vi "re_ClientSrv Tree Controller.vi"(0 "method":T2=enum."initialize", 5 "start path":path, 7 "tree control reference":refnum<vi>, 9 "pattern":string, 11 "file manipulation (local)":T1) -> ()   [LabVIEW 2012]
doc: "Initialises and populates a tree control with local or remote files and directories. This VI is reentrant so as to allow for parallel update of trees. The tags of each tree entry correspond to the path of the file or directory surrounded by double quotes."
uses:
  typedefs/t_ClientSrv Tree Controller Methods.ctl
  served/ClientSrv Server File Manipulation_srv.ctl
  typedefs/t_ClientSrv Tree Controller States.ctl
  typedefs/t_ClientSrv Server File Manipulation Methods.ctl
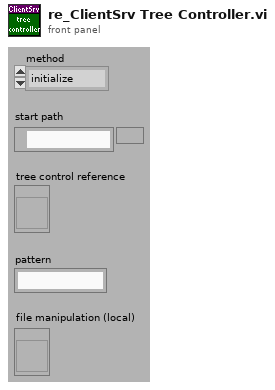
[diagram p1: front panel]
types:
  T1 = typedef "ClientSrv Server File Manipulation_srv.ctl" = refnum<vi>
  T2 = typedef "t_ClientSrv Tree Controller Methods.ctl" = enum16{"do nothing", "initialize", "open item", "close item", "refresh"}
  T3 = typedef "t_ClientSrv Tree Controller States.ctl" = enum16{"initialize", "init roots", "reinit roots", "open item", "close item", "populate", "readjust", "refresh", "stop"}
  T4 = typedef "t_ClientSrv Server File Manipulation Methods.ctl" = enum16{"close", "list", "open", "new", "read", "write", "newdir", "info", "rename", "delete"}
  T5 = typedef "LVNodeAndColumnTypeDef.ctl" = cluster{"Node":string, "Column":i32}
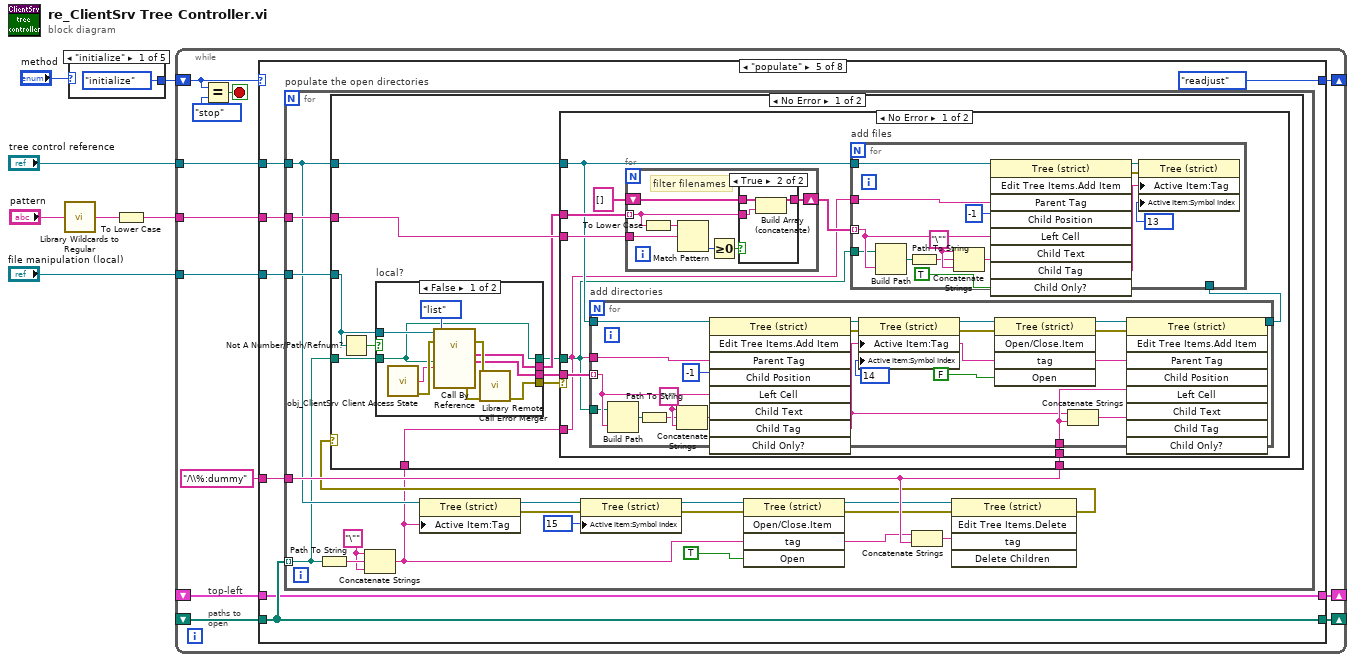
[diagram p0: block diagram]
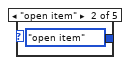
[diagram p2: hidden frame]
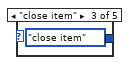
[diagram p3: hidden frame]
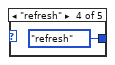
[diagram p4: hidden frame]
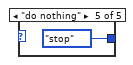
[diagram p5: hidden frame]
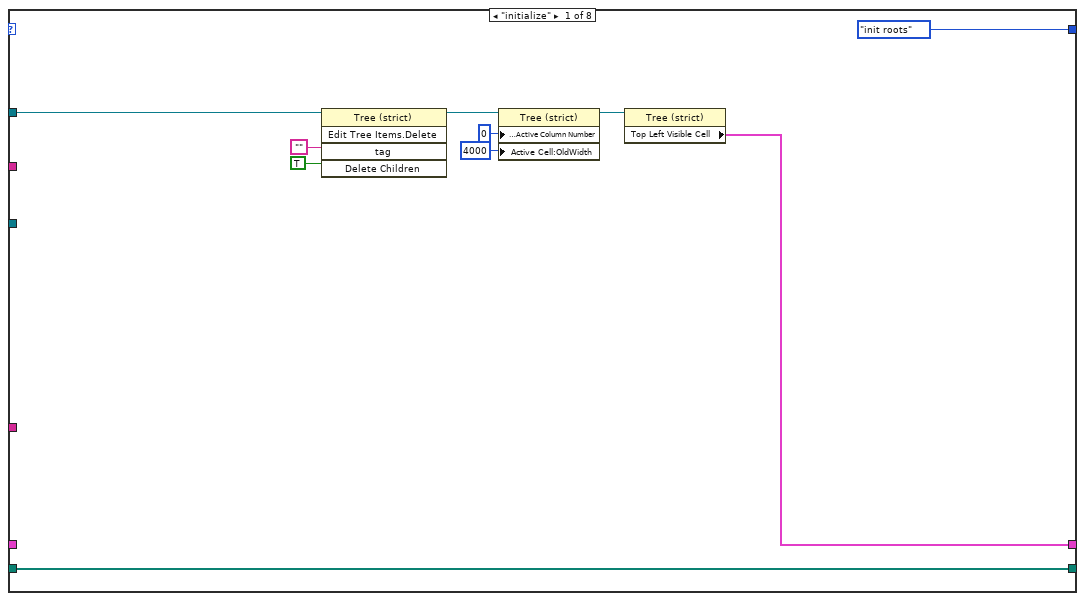
[diagram p6: hidden frame]
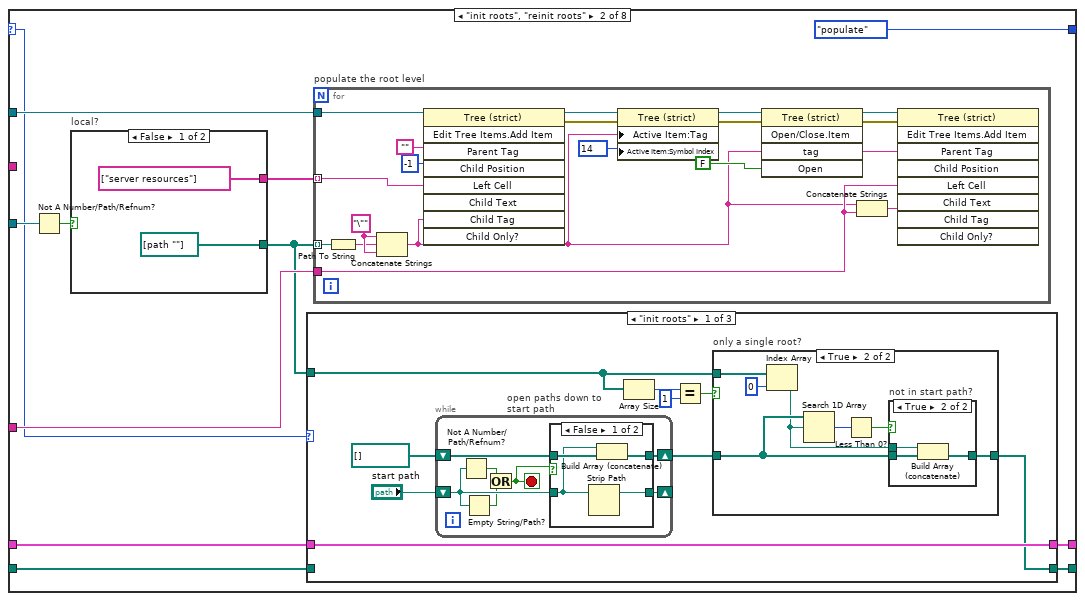
[diagram p7: hidden frame]
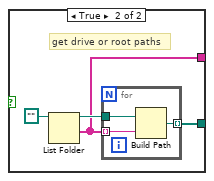
[diagram p13: hidden frame]
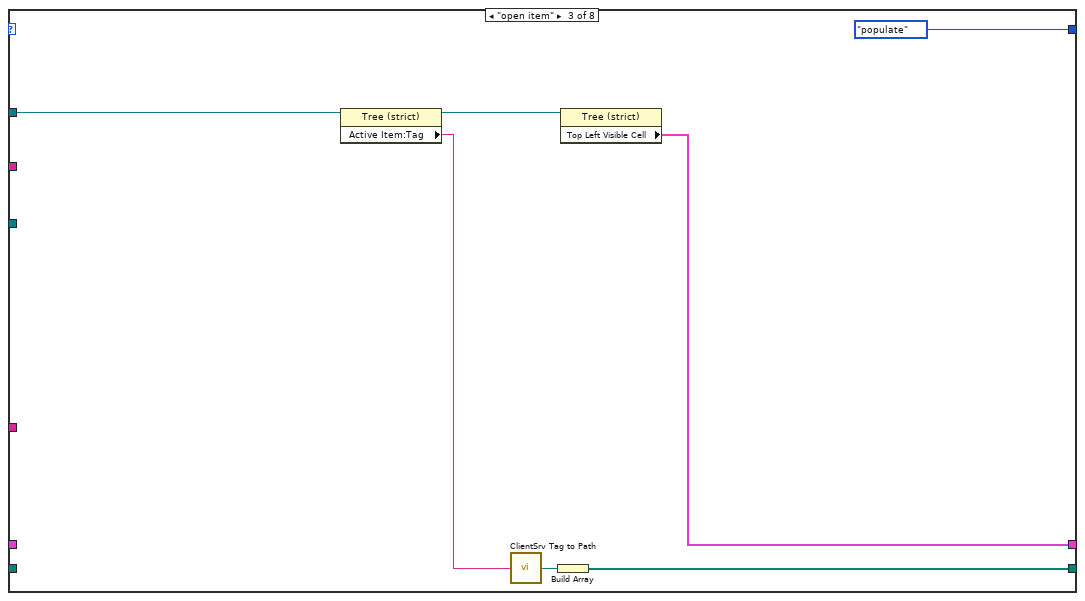
[diagram p14: hidden frame]
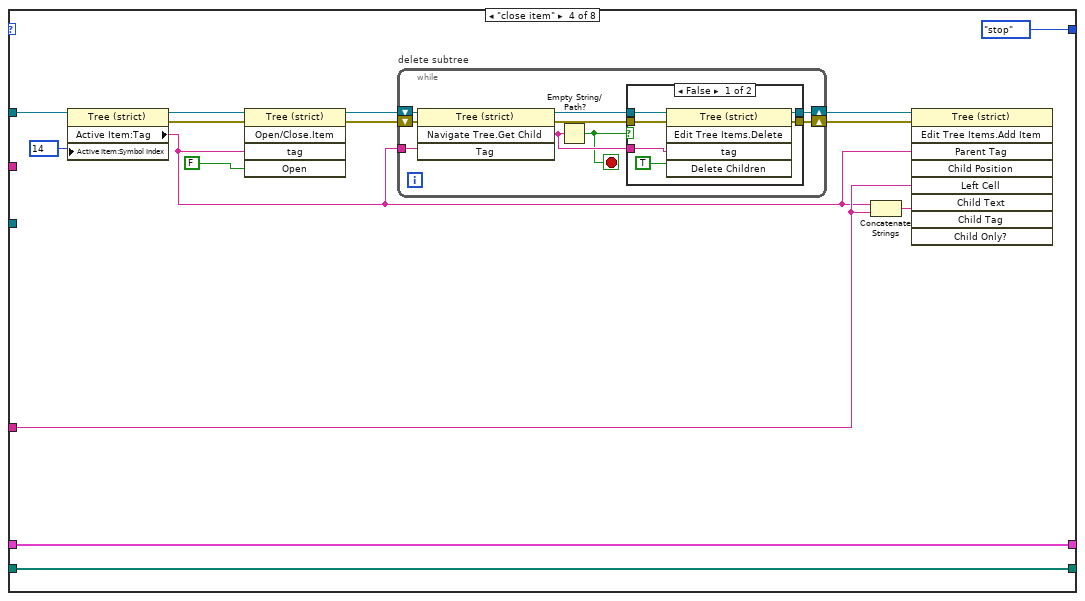
[diagram p15: hidden frame]
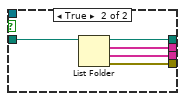
[diagram p17: hidden frame]
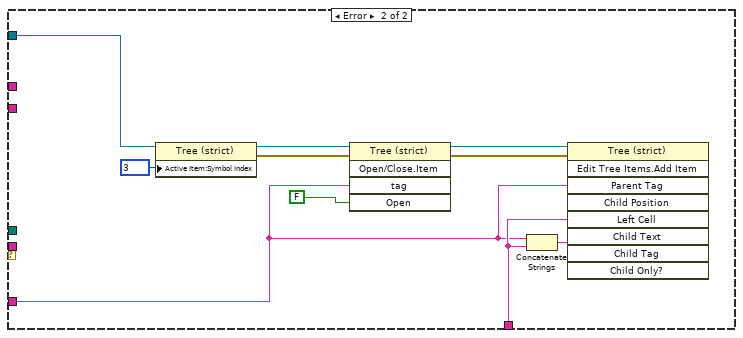
[diagram p19: hidden frame]
diagram:
  n1 = call "Library Wildcards to Regular.vi"("wildcards"="pattern") -> ("regular expression"=w1:string)  [unwired: 4 in]
  n2 = case shown="\"initialize\"" "method" {
    tunnel: [t_ClientSrv_Tree_Controller_States."initialize" ("y") t_ClientSrv_Tree_Controller_States."open item" ("y") t_ClientSrv_Tree_Controller_States."close item" ("y") t_ClientSrv_Tree_Controller_States."refresh" ("y") t_ClientSrv_Tree_Controller_States."stop" ("y")] -> w4
    frame "initialize" {
    }
    frame "open item" {
    }
    frame "close item" {
    }
    frame "refresh" {
    }
    frame "do nothing" {
    }
  }
  n3 = To Lower Case(string=w1) -> (all lower case string=w3:string)
  n4 = while {
    shift-right: [w24] -> _
    shift-left: _ -> [w23]
    shift-right: [w22] -> _
    shift-left: _ -> [w21]
    shift-right: [w17] -> _
    shift-left: w4 -> [w18]
    tunnel: w3 -> [w16]
    tunnel: "tree control reference" -> [w15]
    tunnel: "file manipulation (local)" -> [w13]
    stop <- w19 stop-if-true
    # "top-left"
    # "paths to open"
    n5 = Equal?(x=w18, y=t_ClientSrv_Tree_Controller_States."stop") -> (x = y?=w19:bool)
    n6 = case shown="\"populate\"" w18 {
      selector: w18 -> [_ w35 _ _ _ _ _ w330]
      tunnel: w16 -> [_ _ _ _ w157 _ _ _]
      tunnel: w15 -> [w34 w46 w118 w130 w156 w271 w280 _]
      tunnel: [w26 w38 w117 w132 w153 w272 w286 w331] -> w22
      tunnel: [w28 w40 w115 w133 w155 w274 w283 w332] -> w24
      tunnel: w23 -> [w28 w37 _ w133 w155 w274 _ w332]
      tunnel: w21 -> [_ w39 _ w132 w153 w272 _ w331]
      tunnel: [t_ClientSrv_Tree_Controller_States."init roots" ("y") t_ClientSrv_Tree_Controller_States."populate" ("y") t_ClientSrv_Tree_Controller_States."populate" ("y") t_ClientSrv_Tree_Controller_States."stop" ("y") t_ClientSrv_Tree_Controller_States."readjust" ("y") t_ClientSrv_Tree_Controller_States."stop" ("y") t_ClientSrv_Tree_Controller_States."reinit roots" ("y") w330] -> w17
      tunnel: "/\\%:dummy" ("Left Cell String") -> [_ w41 _ w127 w152 _ _ _]
      tunnel: w13 -> [_ w44 _ _ w151 _ _ _]
      frame "initialize" {
        n7 = invoke on="Invoke Node" class="Tree (strict)" method="Edit Tree Items.Delete"(reference=w34, "tag"="", "Delete Children"=TRUE) -> (reference out=w25:refnum<vi>)  [unwired: 2 in, 4 out]
        n8 = property on="Property Node" class="Tree (strict)"(reference=w25, "Active Cell:Active Column Number"=0 ("Active Cell Properties:Active Column Number"), "Active Cell:OldWidth"=4000 ("Active Cell Properties:Cell Size:Width")) -> (reference out=w27:refnum<vi>)  [unwired: 1 in, 1 out]
        n9 = property on="Property Node" class="Tree (strict)"(reference=w27) -> ("Top Left Visible Cell"=w26:T5)  [unwired: 1 in, 2 out]
      }
      frame "init roots", "reinit roots" {
        n10 = Not A Number/Path/Refnum?(number/path/refnum=w44) -> (NaN/Path/Refnum?=w42:bool)
        n11 = case "local?" shown="False" w42 {
          tunnel: [path[] [path ""] w88] -> w36
          tunnel: [string[] ["server resources"] w87] -> w43
          frame False {
          }
          frame True {
            # "get drive or root paths"
            n12 = List Folder(path=path "") -> (path out=w90:path, folder names=w87:string[])  [unwired: 3 in, 2 out]
            n13 = for {
              tunnel: w90 -> [w93]
              tunnel: w87 -> [w91] mode=indexing
              tunnel: [w92] -> w88 mode=indexing
              n14 = Build Path(base path=w93, name or relative path=w91) -> (appended path=w92:path)
            }
          }
        }
        n15 = case shown="\"init roots\"" w35 {
          tunnel: [w48 w81 w83] -> w40
          tunnel: w39 -> [w52 w82 w84]
          tunnel: [w52 w82 w84] -> w38
          tunnel: w37 -> [_ w81 w83]
          tunnel: w36 -> [w51 _ _]
          frame "init roots" {
            n16 = while "open paths down to start path" {
              shift-right: [w62] -> _
              shift-left: "start path" -> [w59]
              shift-right: [w60] -> w49
              shift-left: path[] [] -> [w61]
              stop <- w56 stop-if-true
              n17 = Not A Number/Path/Refnum?(number/path/refnum=w59) -> (NaN/Path/Refnum?=w58:bool)
              n18 = Empty String/Path?(string/path=w59) -> (empty?=w57:bool)
              n19 = Or(x=w58, y=w57) -> (x .or. y?=w56:bool)
              n20 = case shown="False" w56 {
                tunnel: w59 -> [w64 w68]
                tunnel: [w66 w68] -> w62
                tunnel: w61 -> [w65 w67]
                tunnel: [w63 w67] -> w60
                frame False {
                  n21 = Strip Path(path=w64) -> (stripped path=w66:path)  [unwired: 1 out]
                  n22 = Build Array (concatenate)(w64, w65) -> (w63:path[])
                }
                frame True {
                }
              }
            }
            n23 = Array Size(array=w51) -> (size(s)=w55:i32)
            n24 = Equal?(x=w55, y=1) -> (x = y?=w53:bool)
            n25 = case "only a single root?" shown="True" w53 {
              tunnel: w51 -> [_ w76]
              tunnel: w49 -> [w69 w72]
              tunnel: [w69 w71] -> w48
              frame False {
              }
              frame True {
                n26 = Index Array(array=w76, index=0) -> (element=w70:path)
                n27 = Search 1D Array(1D array=w72, element=w70) -> (index of element=w74:i32)  [unwired: 1 in]
                n28 = Less Than 0?(x=w74) -> (x < 0?=w73:bool)
                n29 = case "not in start path?" shown="True" w73 {
                  tunnel: w72 -> [w77 w80]
                  tunnel: [w77 w79] -> w71
                  tunnel: w70 -> [_ w78]
                  frame False {
                  }
                  frame True {
                    n30 = Build Array (concatenate)(w78, w80) -> (w79:path[])
                  }
                }
              }
            }
          }
          frame "reinit roots" {
          }
          frame Default {
            # "never happens"
          }
        }
        n31 = for "populate the root level" {
          tunnel: w46 -> [w111]
          tunnel: w36 -> [w95] mode=indexing
          tunnel: w43 -> [w101] mode=indexing
          tunnel: w41 -> [w99]
          w97 = "\"" ("string")
          n32 = Path To String(path=w95) -> (string=w96:string)
          n33 = Concatenate Strings(w97, w96, w97) -> (w94:string)
          n34 = invoke class="Tree (strict)" method="Edit Tree Items.Add Item"(reference=w111, "Parent Tag"="", "Child Position"=-1, "Left Cell"=w101, "Child Tag"=w94) -> (reference out=w110:refnum<vi>, error out=w108:errorcluster)  [unwired: 4 in, 7 out]
          n35 = property class="Tree (strict)"(reference=w110, error in=w108, "Active Item:Tag"=w94, "Active Item:Symbol Index"=14) -> (reference out=w107:refnum<vi>, error out=w106:errorcluster)
          n36 = invoke class="Tree (strict)" method="Open/Close.Item"(reference=w107, error in=w106, "tag"=w94, "Open"=FALSE) -> (reference out=w105:refnum<vi>, error out=w104:errorcluster)  [unwired: 1 in, 3 out]
          n37 = Concatenate Strings(w94, w99) -> (w103:string)
          n38 = invoke class="Tree (strict)" method="Edit Tree Items.Add Item"(reference=w105, error in=w104, "Parent Tag"=w94, "Left Cell"=w99, "Child Tag"=w103) -> ()  [unwired: 4 in, 9 out]
        }
      }
      frame "open item" {
        n39 = property on="Property Node" class="Tree (strict)"(reference=w118) -> (reference out=w112:refnum<vi>, "Active Item:Tag"=w113:string)  [unwired: 1 in, 1 out]
        n40 = call "ClientSrv Tag to Path.vi"("tree tag"=w113) -> ("path"=w114:path)
        n41 = Build Array(w114) -> (w115:path[])
        n42 = property on="Property Node" class="Tree (strict)"(reference=w112) -> ("Top Left Visible Cell"=w117:T5)  [unwired: 1 in, 2 out]
      }
      frame "close item" {
        n43 = property class="Tree (strict)"(reference=w130, "Active Item:Symbol Index"=14) -> (reference out=w124:refnum<vi>, error out=w121:errorcluster, "Active Item:Tag"=w120:string)  [unwired: 1 in]
        n44 = invoke on="Invoke Node" class="Tree (strict)" method="Open/Close.Item"(reference=w124, error in=w121, "tag"=w120, "Open"=FALSE) -> (reference out=w123:refnum<vi>, error out=w122:errorcluster)  [unwired: 1 in, 3 out]
        n45 = while "delete subtree" {
          tunnel: w120 -> [w141]
          shift-right: [w137] -> w129
          shift-left: w123 -> [w142]
          shift-right: [w134] -> w125
          shift-left: w122 -> [w136]
          stop <- w138 stop-if-true
          n46 = invoke on="Invoke Node" class="Tree (strict)" method="Navigate Tree.Get Child"(reference=w142, error in=w136, "Tag"=w141) -> (reference out=w140:refnum<vi>, error out=w135:errorcluster, "Navigate Tree:Get Child"=w139:string)  [unwired: 1 in, 1 out]
          n47 = Empty String/Path?(string/path=w139) -> (empty?=w138:bool)
          n48 = case shown="False" w138 {
            tunnel: w140 -> [w148 w150]
            tunnel: w139 -> [w147 _]
            tunnel: [w145 w150] -> w137
            tunnel: w135 -> [w144 w149]
            tunnel: [w143 w149] -> w134
            frame False {
              n49 = invoke on="Invoke Node" class="Tree (strict)" method="Edit Tree Items.Delete"(reference=w148, error in=w144, "tag"=w147, "Delete Children"=TRUE) -> (reference out=w145:refnum<vi>, error out=w143:errorcluster)  [unwired: 1 in, 3 out]
            }
            frame True {
            }
          }
        }
        n50 = Concatenate Strings(w120, w127) -> (w128:string)
        n51 = invoke class="Tree (strict)" method="Edit Tree Items.Add Item"(reference=w129, error in=w125, "Parent Tag"=w120, "Left Cell"=w127, "Child Tag"=w128) -> ()  [unwired: 4 in, 9 out]
      }
      frame "populate" {
        n52 = for "populate the open directories" {
          tunnel: w155 -> [w160] mode=indexing
          tunnel: w157 -> [w175]
          tunnel: w156 -> [w167]
          tunnel: w152 -> [w174]
          tunnel: w151 -> [w173]
          w161 = "\"" ("string")
          n53 = Path To String(path=w160) -> (string=w162:string)
          n54 = Concatenate Strings(w161, w162, w161) -> (w159:string)
          n55 = property on="Property Node" class="Tree (strict)"(reference=w167, "Active Item:Tag"=w159) -> (reference out=w166:refnum<vi>, error out=w158:errorcluster)  [unwired: 1 in]
          n56 = property on="Property Node" class="Tree (strict)"(reference=w166, error in=w158, "Active Item:Symbol Index"=15) -> (reference out=w165:refnum<vi>, error out=w164:errorcluster)
          n57 = invoke on="Invoke Node" class="Tree (strict)" method="Open/Close.Item"(reference=w165, error in=w164, "tag"=w159, "Open"=TRUE ("Delete Children")) -> (reference out=w172:refnum<vi>, error out=w169:errorcluster)  [unwired: 1 in, 3 out]
          n58 = Concatenate Strings(w159, w174) -> (w171:string)
          n59 = invoke on="Invoke Node" class="Tree (strict)" method="Edit Tree Items.Delete"(reference=w172, error in=w169, "tag"=w171) -> (error out=w168:errorcluster)  [unwired: 2 in, 4 out]
          n60 = case shown="No Error" w168 {
            tunnel: w160 -> [w186 _]
            tunnel: w175 -> [w185 _]
            tunnel: w167 -> [w184 _]
            tunnel: w174 -> [w183 _]
            tunnel: w173 -> [w181 _]
            tunnel: w159 -> [w176 _]
            frame No Error {
              n61 = Not A Number/Path/Refnum?(number/path/refnum=w181) -> (NaN/Path/Refnum?=w182:bool)
              n62 = case "local?" shown="False" w182 {
                tunnel: w186 -> [w192 w201]
                tunnel: [w191 w200] -> w180
                tunnel: [w188 w199] -> w179
                tunnel: [w187 w198] -> w178
                tunnel: [w192 w197] -> w177
                tunnel: w181 -> [w195 _]
                frame False {
                  n63 = call "obj_ClientSrv Client Access State.vi"() -> ("certificate"=w193:string, "error out"=w196:errorcluster)  [unwired: 14 in]
                  n64 = call-by-ref "?"(reference=w195, error in=w196, "method"=t_ClientSrv_Server_File_Manipulation_Methods."list", "path"=w192, "certificate"=w193) -> (error out=w190:errorcluster, "file names"=w188:string[], "directory names"=w187:string[], 15:"error out"=w189:errorcluster)  [unwired: 5 in, 6 out]
                  n65 = call "Library Remote Call Error Merger.vi"("call by reference node error"=w190, "called VI error (no error)"=w189) -> ("error out"=w191:errorcluster)  [unwired: 13 in]
                }
                frame True {
                  n66 = List Folder(path=w201) -> (path out=w197:path, filenames=w199:string[], folder names=w198:string[], error out=w200:errorcluster)  [unwired: 3 in]
                }
              }
              n67 = case shown="No Error" w180 {
                tunnel: w178 -> [w211 _]
                tunnel: w177 -> [w203 _]
                tunnel: w184 -> [w205 w265]
                tunnel: w185 -> [w207 _]
                tunnel: w179 -> [w209 _]
                tunnel: w183 -> [w204 w258]
                tunnel: w176 -> [w202 w256]
                frame No Error {
                  n68 = for "add directories" {
                    tunnel: w203 -> [w244]
                    tunnel: w211 -> [w254] mode=indexing
                    tunnel: w205 -> [w251]
                    tunnel: [w242] -> w206
                    tunnel: w204 -> [w241]
                    tunnel: w202 -> [w236]
                    w240 = "\"" ("string")
                    n69 = Build Path(base path=w244, name or relative path=w254) -> (appended path=w237:path)
                    n70 = Path To String(path=w237) -> (string=w238:string)
                    n71 = Concatenate Strings(w240, w238, w240) -> (w239:string)
                    n72 = invoke on="Invoke Node" class="Tree (strict)" method="Edit Tree Items.Add Item"(reference=w251, "Parent Tag"=w236, "Child Position"=-1 ("Child Posn"), "Left Cell"=w254, "Child Tag"=w239) -> (reference out=w250:refnum<vi>, error out=w252:errorcluster)  [unwired: 4 in, 7 out]
                    n73 = property on="Property Node" class="Tree (strict)"(reference=w250, error in=w252, "Active Item:Tag"=w239, "Active Item:Symbol Index"=14) -> (reference out=w249:refnum<vi>, error out=w243:errorcluster)
                    n74 = invoke class="Tree (strict)" method="Open/Close.Item"(reference=w249, error in=w243, "tag"=w239, "Open"=FALSE) -> (reference out=w247:refnum<vi>, error out=w246:errorcluster)  [unwired: 1 in, 3 out]
                    n75 = Concatenate Strings(w239, w241) -> (w245:string)
                    n76 = invoke class="Tree (strict)" method="Edit Tree Items.Add Item"(reference=w247, error in=w246, "Parent Tag"=w239, "Left Cell"=w241, "Child Tag"=w245) -> (reference out=w242:refnum<vi>)  [unwired: 4 in, 8 out]
                  }
                  n77 = for {
                    tunnel: w209 -> [w216] mode=indexing
                    shift-right: [w214] -> w208
                    shift-left: string[] [] -> [w215]
                    tunnel: w207 -> [w213]
                    # "filter filenames"
                    n78 = To Lower Case(string=w216) -> (all lower case string=w212:string)
                    n79 = Match Pattern(string=w212, regular expression=w213) -> (offset past match=w218:i32)  [unwired: 1 in, 3 out]
                    n80 = Greater Or Equal To 0?(x=w218) -> (x >= 0?=w217:bool)
                    n81 = case shown="True" w217 {
                      tunnel: w216 -> [_ w222]
                      tunnel: w215 -> [w219 w221]
                      tunnel: [w219 w220] -> w214
                      frame False {
                      }
                      frame True {
                        n82 = Build Array (concatenate)(w221, w222) -> (w220:string[])
                      }
                    }
                  }
                  n83 = for "add files" {
                    tunnel: w203 -> [w232]
                    tunnel: w208 -> [w234] mode=indexing
                    tunnel: w205 -> [w229]
                    tunnel: w206 -> [_]
                    tunnel: w202 -> [w223]
                    w227 = "\"" ("string")
                    n84 = Build Path(base path=w232, name or relative path=w234) -> (appended path=w225:path)
                    n85 = Path To String(path=w225) -> (string=w226:string)
                    n86 = Concatenate Strings(w227, w226, w227) -> (w224:string)
                    n87 = invoke on="Invoke Node" class="Tree (strict)" method="Edit Tree Items.Add Item"(reference=w229, "Parent Tag"=w223, "Child Position"=-1 ("Child Posn"), "Left Cell"=w234, "Child Tag"=w224, "Child Only?"=TRUE) -> (reference out=w228:refnum<vi>, error out=w231:errorcluster)  [unwired: 3 in, 7 out]
                    n88 = property on="Property Node" class="Tree (strict)"(reference=w228, error in=w231, "Active Item:Tag"=w224, "Active Item:Symbol Index"=13) -> ()  [unwired: 2 out]
                  }
                }
                frame Error {
                  n89 = property on="Property Node" class="Tree (strict)"(reference=w265, "Active Item:Symbol Index"=3) -> (reference out=w263:refnum<vi>, error out=w262:errorcluster)  [unwired: 1 in]
                  n90 = invoke on="Invoke Node" class="Tree (strict)" method="Open/Close.Item"(reference=w263, error in=w262, "tag"=w256, "Open"=FALSE) -> (reference out=w259:refnum<vi>, error out=w257:errorcluster)  [unwired: 1 in, 3 out]
                  n91 = Concatenate Strings(w256, w258) -> (w260:string)
                  n92 = invoke class="Tree (strict)" method="Edit Tree Items.Add Item"(reference=w259, error in=w257, "Parent Tag"=w256, "Left Cell"=w258, "Child Tag"=w260) -> ()  [unwired: 4 in, 9 out]
                }
              }
            }
            frame Error {
            }
          }
        }
      }
      frame "readjust" {
        n93 = property on="Property Node" class="Tree (strict)"(reference=w271) -> (reference out=w270:refnum<vi>, "Value"=w269:string)  [unwired: 1 in, 1 out]
        n94 = property on="Property Node" class="Tree (strict)"(reference=w270, "Active Item:Tag"=w269) -> (reference out=w267:refnum<vi>, error out=w268:errorcluster)  [unwired: 1 in]
        n95 = case "selected item still present?" shown="Error" w268 {
          tunnel: w267 -> [w275 w278]
          tunnel: [w275 w277] -> w266
          frame No Error {
          }
          frame Error {
            n96 = property on="Property Node" class="Tree (strict)"(reference=w278, "Value"="") -> (reference out=w277:refnum<vi>)  [unwired: 1 in, 1 out]
          }
        }
        n97 = property on="Property Node" class="Tree (strict)"(reference=w266, "Top Left Visible Cell"=w272) -> ()  [unwired: 1 in, 2 out]
      }
      frame "refresh" {
        w287 = string[] []
        n98 = property on="Property Node" class="Tree (strict)"(reference=w280) -> (reference out=w285:refnum<vi>, "Top Left Visible Cell"=w286:T5)  [unwired: 1 in, 1 out]
        n99 = while "traverse tree breadth-first to determine the open directories" {
          shift-right: [w298] -> _
          shift-left: "" -> [w293]
          shift-right: [w305] -> w284
          shift-left: w287 -> [w306]
          shift-right: [w303] -> _
          shift-left: w287 -> [w304]
          shift-right: [w297] -> w281
          shift-left: w285 -> [w297]
          stop <- w299 stop-if-true
          # "open directories to traverse"
          # "open directories"
          n100 = property on="Property Node" class="Tree (strict)"(reference=w297, "Active Item:Tag"=w293) -> (reference out=w296:refnum<vi>, "Active Item:Open?"=w294:bool, "Active Item:Child-Only?"=w295:bool)  [unwired: 1 in, 1 out]
          n101 = Empty String/Path?(string/path=w293) -> (empty?=w291:bool)
          n102 = Compound Arithmetic op=AND(w294, invert w295, invert w291) -> (w292:bool)
          n103 = case "open directory?" shown="False" w292 {
            tunnel: w306 -> [w313 w329]
            tunnel: w293 -> [w311 w325]
            tunnel: [w313 w328] -> w305
            tunnel: w304 -> [w312 w327]
            tunnel: [w310 w324] -> w298
            tunnel: [w309 w326] -> w303
            tunnel: w296 -> [w308 w323]
            tunnel: w291 -> [w307 _]
            frame False {
              n104 = case shown="True" w307 {
                tunnel: w312 -> [w317 w322]
                tunnel: [w315 w320] -> w310
                tunnel: [w317 w319] -> w309
                tunnel: w311 -> [w316 _]
                tunnel: w308 -> [w314 w318]
                frame False {
                  n105 = invoke on="Invoke Node" class="Tree (strict)" method="Navigate Tree.Get Next"(reference=w314, "Tag"=w316) -> ("Navigate Tree:Get Next Item"=w315:string)  [unwired: 2 in, 3 out]
                }
                frame True {
                  n106 = Delete From Array(array=w322) -> (deleted portion=w321:string, array with subset deleted=w319:string[])  [unwired: 2 in]
                  n107 = invoke on="Invoke Node" class="Tree (strict)" method="Navigate Tree.Get Child"(reference=w318, "Tag"=w321) -> ("Navigate Tree:Get Child"=w320:string)  [unwired: 2 in, 3 out]
                }
              }
            }
            frame True {
              n108 = Build Array (concatenate)(w329, w325) -> (w328:string[])
              n109 = Build Array (concatenate)(w327, w325) -> (w326:string[])
              n110 = invoke on="Invoke Node" class="Tree (strict)" method="Navigate Tree.Get Next"(reference=w323, "Tag"=w325) -> ("Navigate Tree:Get Next Item"=w324:string)  [unwired: 2 in, 3 out]
            }
          }
          n111 = Array Size(array=w303) -> (size(s)=w302:i32)
          n112 = Empty String/Path?(string/path=w298) -> (empty?=w300:bool)
          n113 = Equal To 0?(x=w302) -> (x = 0?=w301:bool)
          n114 = And(x=w300, y=w301) -> (x .and. y?=w299:bool)
        }
        n115 = invoke on="Invoke Node" class="Tree (strict)" method="Edit Tree Items.Delete"(reference=w281, "Delete Children"=TRUE) -> ()  [unwired: 3 in, 5 out]
        n116 = for {
          tunnel: w284 -> [w290] mode=indexing
          tunnel: [w289] -> w283 mode=indexing
          n117 = call "ClientSrv Tag to Path.vi"("tree tag"=w290) -> ("path"=w289:path)
        }
      }
      frame "stop" {
      }
    }
  }
